vi "WSVCAP SHL FPGA LL SPI_RFFE Load Next Cycle CMD.vi"(0 "Transfer Cluster In":T1={"Transaction"=enum."I2C-Read Data", "Write Byte"=0, "Write Bits Remaining"=3, "Read Bits Remaining"=0, "Read Bytes Remaining"=0, "Wait Ticks Remaining"=0, "Slave Address"=0, "Bytes to Read"=2, "Bytes to Write"=0, "Sub Address"=0, "Socket Mask"=0, "Write CMD [1-4]"=2, "Write Bit Index [0-18]"=2, "CMD Delay (Ticks)"=7, "Commands per Cycle [1-4]"=8, "CMD Length [1-48]"=0, "Cycle Count"=1, "Cycle Mode"=TRUE, "CMD 1 Length (Bits)"=0, "CMD 2 Length (Bits)"=0, "CMD 3 Length (Bits)"=0, "CMD 4 Length (Bits)"=0, "CMD 1 Delay (Ticks)"=0, "CMD 2 Delay (Ticks)"=0, "CMD 3 Delay (Ticks)"=2, "CMD 4 Delay (Ticks)"=2, "CMD 1"=0, "CMD 2"=0, "CMD 3"=0, "CMD 4"=0, "Cycle CMD"=0, "Transaction Step"=enum."I2C Write - II:Send Sub Address", "Operation Step"=enum."I2C Send Slave Add - C: Send Address Byte", "Procedure Step"=enum."I2C Start/Stop - 1: Set Clock Low", "Start Operation"=FALSE, "Start Procedure"=FALSE, "Procedure"=enum."I2C-Send Address Byte", "Wait Ticks"=2, "UUT Set (0/1)"=0} {"Cycle CMD" format="%.0x"; "CMD 4" format="%.0x"; "CMD 3" format="%.0x"; "CMD 2" format="%.0x"; "CMD 1" format="%.0x"; "Socket Mask" format="%06x"}) -> (4 "Transfer Cluster Out":T1={"Transaction"=enum."I2C-Read Data", "Write Byte"=0, "Write Bits Remaining"=3, "Read Bits Remaining"=0, "Read Bytes Remaining"=0, "Wait Ticks Remaining"=0, "Slave Address"=0, "Bytes to Read"=2, "Bytes to Write"=0, "Sub Address"=0, "Socket Mask"=0, "Write CMD [1-4]"=2, "Write Bit Index [0-18]"=2, "CMD Delay (Ticks)"=7, "Commands per Cycle [1-4]"=8, "CMD Length [1-48]"=0, "Cycle Count"=1, "Cycle Mode"=TRUE, "CMD 1 Length (Bits)"=0, "CMD 2 Length (Bits)"=0, "CMD 3 Length (Bits)"=0, "CMD 4 Length (Bits)"=0, "CMD 1 Delay (Ticks)"=0, "CMD 2 Delay (Ticks)"=0, "CMD 3 Delay (Ticks)"=2, "CMD 4 Delay (Ticks)"=2, "CMD 1"=0, "CMD 2"=0, "CMD 3"=0, "CMD 4"=0, "Cycle CMD"=0, "Transaction Step"=enum."I2C Write - II:Send Sub Address", "Operation Step"=enum."I2C Send Slave Add - C: Send Address Byte", "Procedure Step"=enum."I2C Start/Stop - 1: Set Clock Low", "Start Operation"=FALSE, "Start Procedure"=FALSE, "Procedure"=enum."I2C-Send Address Byte", "Wait Ticks"=2, "UUT Set (0/1)"=0} {"Cycle CMD" format="%.0x"; "CMD 4" format="%.0x"; "CMD 3" format="%.0x"; "CMD 2" format="%.0x"; "CMD 1" format="%.0x"; "Socket Mask" format="%06x"}, 8 "SPI Cycle Count":u64)   [LabVIEW 2017]
uses:
  Type Defs/WSVCAP SHL Transaction Cluster.ctl
  Type Defs/WSVCAP SHL Transaction Enum.ctl
  Type Defs/WSVCAP SHL Transaction Step Enum.ctl
  Type Defs/WSVCAP SHL Operation Step Enum.ctl
  Type Defs/WSVCAP SHL Procedure Step Enum.ctl
  Type Defs/WSVCAP SHL Procedure Enum.ctl
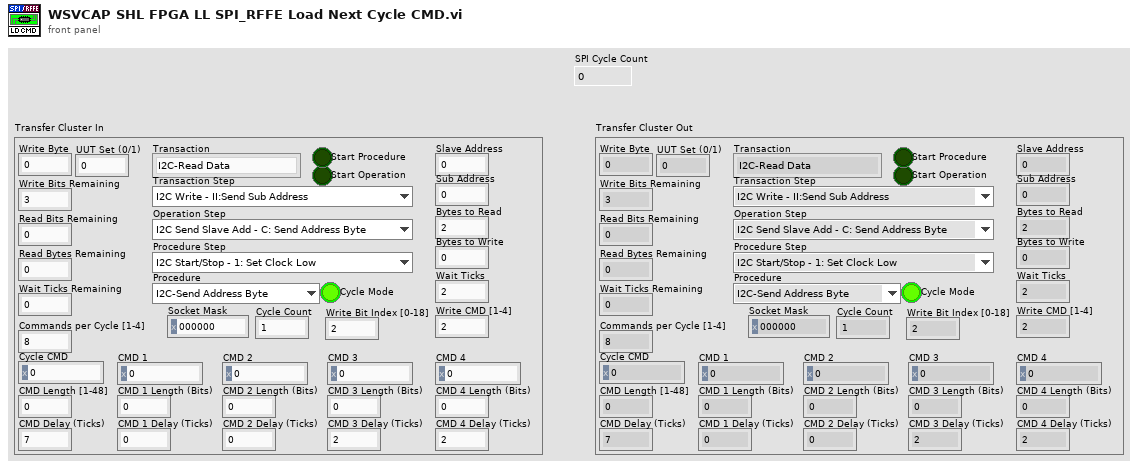
[diagram p1: front panel]
types:
  T1 = typedef "WSVCAP SHL Transaction Cluster.ctl" = cluster{"Transaction":T2, "Write Byte":u8, "Write Bits Remaining":u8, "Read Bits Remaining":u8, "Read Bytes Remaining":u8, "Wait Ticks Remaining":u32, "Slave Address":u8, "Bytes to Read":u8, "Bytes to Write":u8, "Sub Address":u8, "Socket Mask":u32, "Write CMD [1-4]":u8, "Write Bit Index [0-18]":u8, "CMD Delay (Ticks)":u32, "Commands per Cycle [1-4]":u8, "CMD Length [1-48]":u8, "Cycle Count":u64, "Cycle Mode":bool, "CMD 1 Length (Bits)":u8, "CMD 2 Length (Bits)":u8, "CMD 3 Length (Bits)":u8, "CMD 4 Length (Bits)":u8, "CMD 1 Delay (Ticks)":u32, "CMD 2 Delay (Ticks)":u32, "CMD 3 Delay (Ticks)":u32, "CMD 4 Delay (Ticks)":u32, "CMD 1":u64, "CMD 2":u64, "CMD 3":u64, "CMD 4":u64, "Cycle CMD":u64, "Transaction Step":T3, "Operation Step":T4, "Procedure Step":T5, "Start Operation":bool, "Start Procedure":bool, "Procedure":T6, "Wait Ticks":u32, "UUT Set (0/1)":u8}
  T2 = typedef "WSVCAP SHL Transaction Enum.ctl" = enum16{"I2C-Read Data", "I2C-Write Data", "RFFE-Ext Write", "RFFE-Ext Read", "SRL-Write Data"}
  T3 = typedef "WSVCAP SHL Transaction Step Enum.ctl" = enum16{"I2C Write - I:Send Slave Address", "I2C Write - II:Send Sub Address", "I2C Write - III:Send Data Bytes", "I2C Read - I:Send Slave Address (W)", "I2C Read - II:Send Sub Address", "I2C Read - III:Send Slave Address (R)", "I2C Read - IV:Read Data Bytes", "RFFE Ext Write - I.Write Data", "RFFE Ext Read - I:Read Data", "SRL Write - I:Write Data"}
  T4 = typedef "WSVCAP SHL Operation Step Enum.ctl" = enum16{"I2C Send Slave Add - A: Send Start Sequence", "I2C Send Slave Add - B: Load Address Byte", "I2C Send Slave Add - C: Send Address Byte", "I2C Send Slave Add - D: Read Slave ACK", "I2C Send Sub Add - A: Load Sub Address", "I2C Send Sub Add - B: Send Address Byte", "I2C Send Sub Add - C: Read Slave ACK", "I2C Send Data - A: Get Byte from FIFO", "I2C Send Data - B: Send Data Byte", "I2C Send Data - C: Read Slave ACK", "I2C Send Data - D: Send Stop Sequence", "I2C Read Data - A: Load Bytes to Read", "I2C Read Data - B: Receive Byte", "I2C Read Data - C: Write Master ACK", "I2C Read Data - D: Send Stop Sequence", "RFFE Read Data - A: Send SSC", "RFFE Read Data - B: Send CMD Frame", "RFFE Read Data - C: Receive Byte", "RFFE Write Data - A: Send SSC", "RFFE Write Data - B: Send Data", "RFFE Write Data - C: Wait CMD Delay", "RFFE Write Data - D: Clear Lines", "SRL Write Data - A: Send Data", "SRL Write Data - B: Wait CMD Delay", "SRL Write Data - C: Clear Lines"}
  T5 = typedef "WSVCAP SHL Procedure Step Enum.ctl" = enum16{"I2C Start/Stop - 1: Set Clock Low", "I2C Start/Stop - 2: Wait", "I2C Start/Stop - 3: Set Data I", "I2C Start/Stop - 4: Wait", "I2C Start/Stop - 5: Set Clock High", "I2C Start/Stop - 6: Wait", "I2C Start/Stop - 7: Set Data II", "I2C Start/Stop - 8: Wait", "I2C Start/Stop - 9: Set Clock Low", "I2C Start/Stop - 10: Wait", "I2C Read ACK - 1: Set Clock High", "I2C Read ACK - 2: Wait", "I2C Read ACK - 3: Read ACK Bit", "I2C Read ACK - 4: Wait", "I2C Read ACK - 5: Set Clock Low", "I2C Read ACK - 6: Wait", "I2C Write ACK - 1: Write ACK Bit", "I2C Write ACK - 2: Wait", "I2C Write ACK - 3: Set Clock High", "I2C Write ACK - 4: Wait", "I2C Write ACK - 5: Set Clock Low", "I2C Write ACK - 6: Wait", "I2C Write ACK - 7: Set Data Low", "I2C Send Add - 1: Reset Bits Remaining", "I2C Send Add - 2: Set Data Bit", "I2C Send Add - 3: Wait", "I2C Send Add - 4: Set Clock High", "I2C Send Add - 5: Wait", "I2C Send Add - 6: Set Clock Low", "I2C Send Add - 7: Wait", "I2C Send Add - 8: Check Bits Remaining", "I2C Send Data - 1: Reset Bits Remaining", "I2C Send Data - 2: Load Write Bit from FIFO", "I2C Send Data - 3: Set Data Bit", "I2C Send Data - 4: Wait", "I2C Send Data - 5: Set Clock High", "I2C Send Data - 6: Wait", "I2C Send Data - 7: Set Clock Low", "I2C Send Data - 8: Wait", "I2C Send Data - 9: Check Bits Remaining", "I2C Receive Data - 1: Reset Bits Remaining", "I2C Receive Data - 2: Wait", "I2C Receive Data - 3: Set Clock High", "I2C Receive Data - 4: Wait", "I2C Receive Data - 5: Read Data Bit", "I2C Receive Data - 6: Wait", "I2C Receive Data - 7: Set Clock Low", "I2C Receive Data - 8: Wait", "I2C Receive Data - 9: Check Bits Remaining", "RFFE Send SSC - 1:Set Low", "RFFE Send SSC - 2:Wait", "RFFE Send SSC - 3:Set SDA High", "RFFE Send SSC - 4:Wait", "RFFE Send SSC - 5:Set SDA Low", "RFFE Send SSC - 6:Wait", "RFFE Send Data - 1:Set SCL High", "RFFE Send Data - 2:Wait", "RFFE Send Data - 3:Set SCL Low", "RFFE Send Data - 4:Wait", "RFFE Send Data - 5:Set SCL High (P)", "RFFE Send Data - 6:Wait", "RFFE Send Data - 7:Set SCL Low (P)", "RFFE Send Data - 8:Wait", "RFFE Send Data - 9:Set SCL High (BP)", "RFFE Send Data - 10:Wait", "RFFE Send Data - 11:Set SCL Low (BP)", "RFFE Send Data - 12:Wait", "RFFE Receive Data - 1:Set SCL High", "RFFE Receive Data - 2:Wait", "RFFE Receive Data - 3:Set SCL Low", "RFFE Receive Data - 4:Wait", "RFFE Receive Data - 5:Set SCL High (BP)", "RFFE Receive Data - 6:Wait", "RFFE Receive Data - 7:Set SCL Low (BP)", "RFFE Receive Data - 8:Wait", "RFFE Wait CMD Delay - 1:Wait", "RFFE Clear Lines - 1:Clear", "SRL Write Data - 1:Set SYNC Low", "SRL Write Data - 2:Set SCLK High", "SRL Write Data - 3:Wait", "SRL Write Data - 4:Set SCLK Low", "SRL Write Data - 5:Wait", "SRL Write Data - 6:Set SYNC High", "SRL Wait CMD Delay - 1:Wait", "SRL Clear Lines - 1:Clear"}
  T6 = typedef "WSVCAP SHL Procedure Enum.ctl" = enum16{"None", "I2C-Send Start/Stop Sequence", "I2C-Send Address Byte", "I2C-Send Data Byte", "I2C-Read ACK", "I2C-Receive Byte", "I2C-Write ACK", "RFFE-Clear Lines", "RFFE-Send SSC", "RFFE-Send Data", "RFFE-Receive Data", "RFFE-Wait CMD Delay", "SRL-Clear Lines", "SRL-Send Data", "SRL-Wait CMD Delay"}
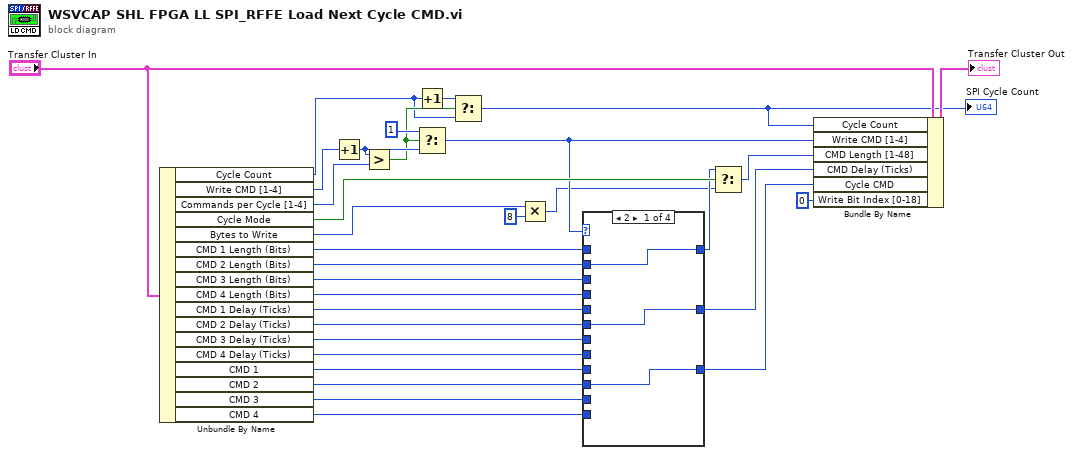
[diagram p0: block diagram]
diagram:
  n1 = Unbundle By Name("Transfer Cluster In") -> ("Cycle Count"=w10:u64, "Write CMD [1-4]"=w27:u8, "Commands per Cycle [1-4]"=w28:u8, "Cycle Mode"=w26:bool, "Bytes to Write"=w2:u8, "CMD 1 Length (Bits)"=w25:u8, "CMD 2 Length (Bits)"=w24:u8, "CMD 3 Length (Bits)"=w23:u8, "CMD 4 Length (Bits)"=w22:u8, "CMD 1 Delay (Ticks)"=w21:u32, "CMD 2 Delay (Ticks)"=w20:u32, "CMD 3 Delay (Ticks)"=w19:u32, "CMD 4 Delay (Ticks)"=w18:u32, "CMD 1"=w5:u64, "CMD 2"=w4:u64, "CMD 3"=w7:u64, "CMD 4"=w6:u64)
  n2 = Increment(x=w27) -> (x+1=w29:u8)
  n3 = Greater?(x=w29, y=w28) -> (0:w11:bool)
  n4 = Increment(x=w10) -> (x+1=w12:u64)
  n5 = Select(t=u8 1 ("f"), s=w11, f=w29) -> (s? t:f=w17:u8)
  n6 = Select(t=w12, s=w11, f=w10) -> (s? t:f=w9:u64)
  "SPI Cycle Count" <- w9
  n7 = Multiply(x=w2, y=u8 8) -> (x*y=w1:u8)
  n8 = case shown="2" w17 {
    tunnel: w25 -> [_ _ _ w44]
    tunnel: w24 -> [w35 _ _ _]
    tunnel: w23 -> [_ w38 _ _]
    tunnel: w22 -> [_ _ w41 _]
    tunnel: w21 -> [_ _ _ w43]
    tunnel: w20 -> [w34 _ _ _]
    tunnel: w19 -> [_ w37 _ _]
    tunnel: w18 -> [_ _ w40 _]
    tunnel: [w35 w38 w41 w44] -> w16
    tunnel: [w34 w37 w40 w43] -> w14
    tunnel: [w33 w36 w39 w42] -> w8
    tunnel: w7 -> [_ w36 _ _]
    tunnel: w6 -> [_ _ w39 _]
    tunnel: w5 -> [_ _ _ w42]
    tunnel: w4 -> [w33 _ _ _]
    frame 2 {
    }
    frame 3 {
    }
    frame 4.. {
    }
    frame ..1 {
    }
  }
  n9 = Select(t=w16, s=w26, f=w1) -> (s? t:f=w15:u8)
  n10 = Bundle By Name(cluster="Transfer Cluster In", "Cycle Count"=w9, "Write CMD [1-4]"=w17, "CMD Length [1-48]"=w15, "CMD Delay (Ticks)"=w14, "Cycle CMD"=w8, "Write Bit Index [0-18]"=u8 0 ("Write Bit Index [0-39]")) -> (→"Transfer Cluster Out":T1)
